vi "FTW-Crypto-PublicKeySignature-Sign.vi"(0 "Data":string="Data to encrypt!", 5 "Private Key XML":string, 11 "error in":errorcluster) -> (4 "Hex Encoded Signature":string, 6 "Key Information":string, 15 "error out":errorcluster)   [LabVIEW 2012]
panel:
  # "Inputs"
  # "Outputs"
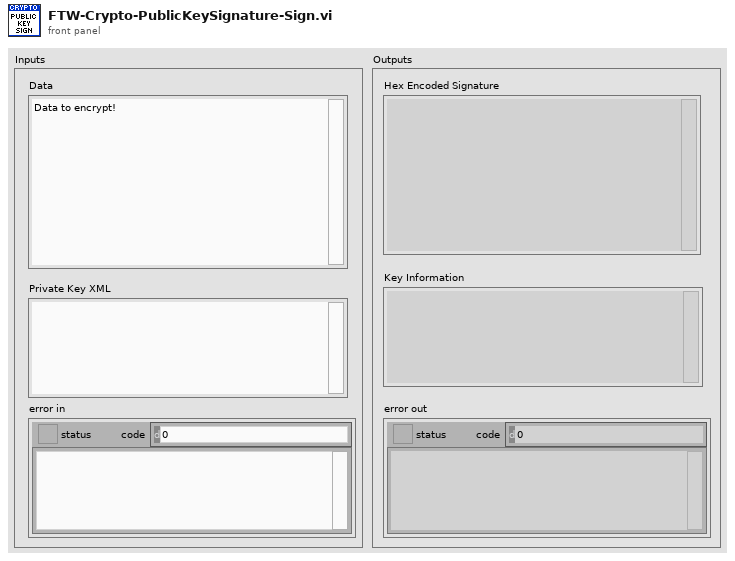
[diagram p1: front panel]
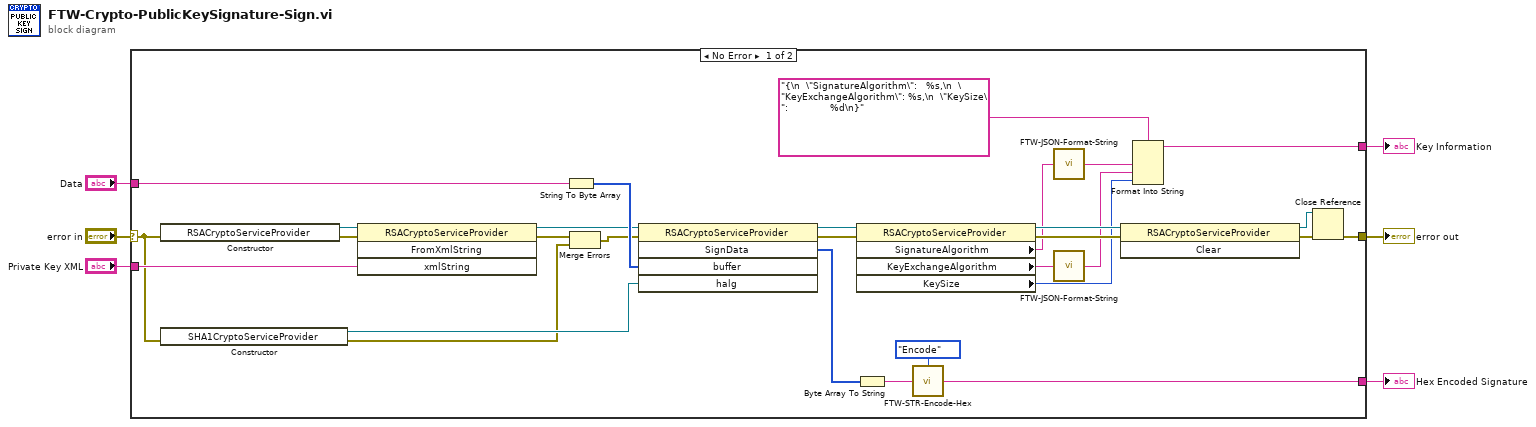
[diagram p0: block diagram]
diagram:
  n1 = case shown="No Error" "error in" {
    selector: "error in" -> [w18 w36]
    tunnel: "Data" -> [w33 _]
    tunnel: [w26 _] -> w5
    tunnel: "Private Key XML" -> [w29 _]
    tunnel: [w35 w36] -> w2
    tunnel: [w12 _] -> w1
    frame No Error {
      n2 = constructor class="RSACryptoServiceProvider"(error in=w18) -> (reference out=w30:refnum<k24>, error out=w31:errorcluster)  [unwired: 2 in, 1 out]
      n3 = constructor class="SHA1CryptoServiceProvider"(error in=w18) -> (reference out=w28:refnum<k24>, error out=w20:errorcluster)  [unwired: 2 in, 1 out]
      n4 = invoke class="RSACryptoServiceProvider" method="FromXmlString"(reference=w30, error in=w31, "xmlString"=w29) -> (reference out=w22:refnum<k24>, error out=w21:errorcluster)  [unwired: 1 in, 2 out]
      n5 = String To Byte Array(string=w33) -> (unsigned byte array=w32:u8[])
      n6 = Merge Errors(w21, w20) -> (w19:errorcluster)
      n7 = invoke class="RSACryptoServiceProvider" method="SignData"(reference=w22, error in=w19, "buffer"=w32, "halg"=w28) -> (reference out=w17:refnum<k24>, error out=w16:errorcluster, "SignData"=w34:u8[])  [unwired: 1 in, 2 out]
      n8 = property class="RSACryptoServiceProvider"(reference=w17, error in=w16) -> (reference out=w15:refnum<k24>, error out=w14:errorcluster, "SignatureAlgorithm"=w10:string, "KeyExchangeAlgorithm"=w7:string, "KeySize"=w11:i32)
      n9 = Byte Array To String(unsigned byte array=w34) -> (string=w27:string)
      n10 = call "FTW-STR-Encode-Hex.vi"("Input"=w27, "Direction"=enum16{"Encode", "Decode"}."Encode") -> ("Output"=w26:string)
      n11 = call "FTW-JSON-Format-String.vi"("LabVIEW String"=w10) -> ("JSON String"=w9:string)
      n12 = call "FTW-JSON-Format-String.vi"("LabVIEW String"=w7) -> ("JSON String"=w8:string)
      n13 = invoke class="RSACryptoServiceProvider" method="Clear"(reference=w15, error in=w14) -> (reference out=w23:refnum<k24>, error out=w24:errorcluster)  [unwired: 1 in, 1 out]
      n14 = Format Into String(format string="{\n  \"SignatureAlgorithm\":   %s,\n  \"KeyExchangeAlgorithm\": %s,\n  \"KeySize\":              %d\n}", w9, w8, w11) -> (resulting string=w12:string)  [unwired: 2 in, 1 out]
      n15 = Close Reference(reference=w23, error in (no error)=w24) -> (error out=w35:errorcluster)
    }
    frame Error {
    }
  }
  "Hex Encoded Signature" <- w5
  "error out" <- w2
  "Key Information" <- w1
